vi "List All.vi"(8 "error in (no error)":errorcluster, 11 "Current Value Table in":refnum<class "Current Value Table.lvclass">) -> (0 "error out":errorcluster, 1 "Variant Attribute":variant, 2 "Tag Names":string[](array[string]), 3 "Current Value Table out":refnum<class "Current Value Table.lvclass">)   [LabVIEW 2024, in "Current Value Table.lvlib" / "Current Value Table.lvclass"]
uses:
  Current Value Table.lvclass
  Current Value Table.lvclass/Current Value Table.ctl
  iCVT_Item/iCVT_Item.lvclass
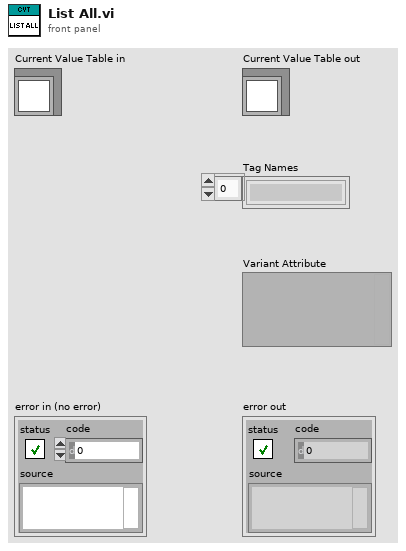
[diagram p1: front panel]
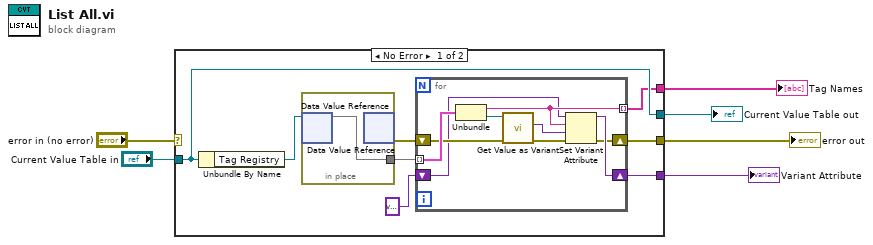
[diagram p0: block diagram]
diagram:
  n1 = case shown="No Error" "error in (no error)" {
    selector: "error in (no error)" -> [_ w26]
    tunnel: [w9 w26] -> w5
    tunnel: [w14 w25] -> w3
    tunnel: "Current Value Table in" -> [w14 w25]
    tunnel: [w11 _] -> w2
    tunnel: [w7 _] -> w1
    frame No Error {
      n2 = Unbundle By Name(w14) -> ("Tag Registry"=w13:refnum<data-value>)
      n3 = in-place {
        in-place-border: [w24] -> w12
        n4 = in-place-dvr #1(w13) -> (w24:map{string, refnum<class "iCVT_Item.lvclass">})  [unwired: 1 out]
        n5 = in-place-dvr #1() -> (w10:errorcluster)  [unwired: 1 in, 1 out]
      }
      n6 = for {
        tunnel: w12 -> [w23] mode=indexing
        tunnel: [w20] -> w11 mode=indexing
        shift-right: [w15] -> w9
        shift-left: w10 -> [w21]
        shift-right: [w17] -> w7
        shift-left: variant -> [w18]
        n7 = Unbundle(w23) -> (w20:string, "Current Value Table.lvlib:iCVT_Item.lvclass"=w22:refnum<class "iCVT_Item.lvclass">)
        n8 = call-dynamic "Get Value as Variant.vi"("error in (no error)"=w21, "iCVT_Item in"=w22) -> ("error out"=w16:errorcluster, "data"=w19:variant)  [unwired: 7 in, 1 out]
        n9 = Set Variant Attribute(Variant=w18, name=w20, value=w19, error in=w16) -> (Variant out=w17:variant, error out=w15:errorcluster)  [unwired: 1 out]
      }
    }
    frame Error {
    }
  }
  "error out" <- w5
  "Current Value Table out" <- w3
  "Tag Names" <- w2
  "Variant Attribute" <- w1
